vi "LockinDAQ.Configure Sweep 2.vi"(8 "error in (no error)":errorcluster, 11 "LockinDAQ in":refnum<class "LockinDAQ.lvclass">) -> (0 "error out":errorcluster, 3 "LockinDAQ out":refnum<class "LockinDAQ.lvclass">)   [LabVIEW 2016, in "LockinDAQ.lvclass"]
uses:
  LockinDAQ.lvclass
  Typedefs/Function-enum.ctl
  LockinDAQ.lvclass/LockinDAQ.ctl
panel:
  out "Frequency (Hz)":dbl
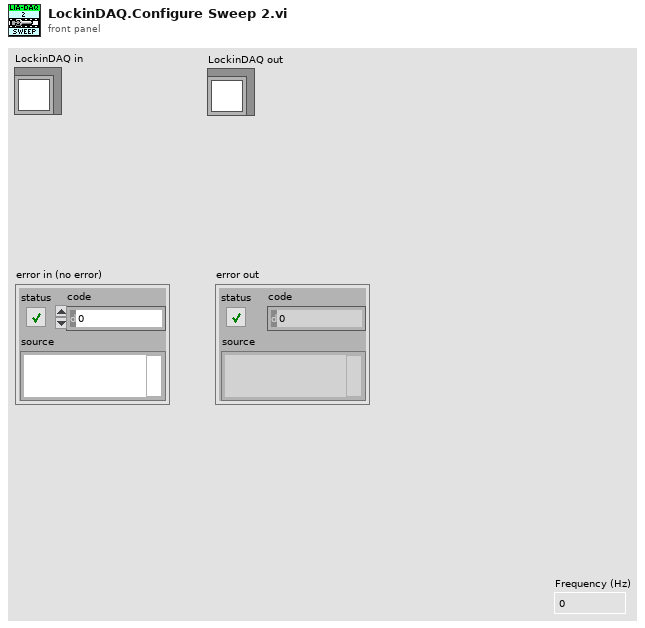
[diagram p1: front panel]
types:
  T1 = typedef "LockinDAQ.lvclass/Function-enum.ctl" = enum16{"Sine", "Triangle", "Square", "Sawtooth"}
  T2 = typedef "LockinDAQ.lvclass/AO-cluster.ctl" = cluster{"AO Amp (V)":T3, "AO DC (V)":T4, "AO f (Hz)":T5, "AO Phase (°)":T6, "Function":T7, "I+":bool[], "Sweeping":bool[]}
  T3 = typedef "LockinDAQ.lvclass/AO_Amp-array.ctl" = dbl[]
  T4 = typedef "LockinDAQ.lvclass/AO_DC-array.ctl" = dbl[]
  T5 = typedef "LockinDAQ.lvclass/AO_f-array.ctl" = dbl[]
  T6 = typedef "LockinDAQ.lvclass/AO_phi-array.ctl" = dbl[]
  T7 = typedef "LockinDAQ.lvclass/Function-array.ctl" = T1[]
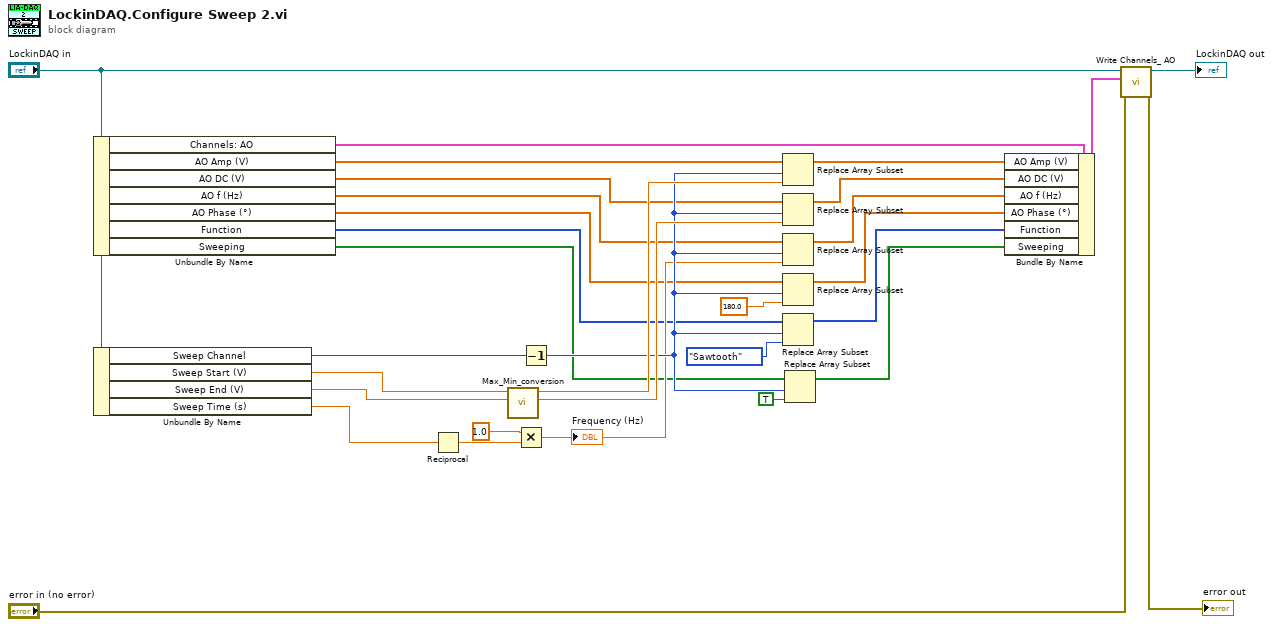
[diagram p0: block diagram]
diagram:
  n1 = Unbundle By Name("LockinDAQ in") -> ("Channels: AO"=w3:T2, "AO Amp (V)"=w18:T3, "AO DC (V)"=w17:T4, "AO f (Hz)"=w16:T5, "AO Phase (°)"=w15:T6, "Function"=w14:T7, "Sweeping"=w13:bool[])
  n2 = Unbundle By Name("LockinDAQ in") -> ("Sweep Channel"=w4:i32, "Sweep Start (V)"=w5:dbl, "Sweep End (V)"=w6:dbl, "Sweep Time (s)"=w1:dbl)
  n3 = Reciprocal(x=w1) -> (1/x=w26:dbl)
  n4 = call <userlib>:"Max_Min_conversion.vi"("Min"=w6, "Max"=w5) -> ("offset"=w24:dbl, "Amplitude"=w25:dbl)  [unwired: 8 in]
  n5 = Multiply(x=1.0, y=w26) -> (x*y=w20:dbl)
  "Frequency (Hz)" <- w20
  n6 = Decrement(x=w4) -> (x-1=w21:i32)
  n7 = Replace Array Subset(array=w18, new element=w25, index=w21) -> (w12:T3)
  n8 = Replace Array Subset(array=w17, new element=w24, index=w21) -> (w11:T4)
  n9 = Replace Array Subset(array=w16, new element=w20, index=w21) -> (w10:T5)
  n10 = Replace Array Subset(array=w15, new element=180.0 ("new element/subarray"), index=w21) -> (w9:T6)
  n11 = Replace Array Subset(array=w14, new element=Function-enum."Sawtooth" ("new element/subarray"), index=w21) -> (w8:T7)
  n12 = Replace Array Subset(array=w13, new element=TRUE ("new element/subarray"), index=w21) -> (w7:bool[])
  n13 = Bundle By Name(cluster=w3, "AO Amp (V)"=w12, "AO DC (V)"=w11, "AO f (Hz)"=w10, "AO Phase (°)"=w9, "Function"=w8, "Sweeping"=w7) -> (w28:T2)
  n14 = call "Write Channels_ AO.vi"("error in (no error)"="error in (no error)", "Channels: AO"=w28, "LockinDAQ"="LockinDAQ in") -> ("error out"=→"error out":errorcluster, "LockinDAQ out"=→"LockinDAQ out":refnum<class "LockinDAQ.lvclass">)  [unwired: 7 in]
